vi "main.vi"() -> ()   [LabVIEW 2018]
uses:
  src/class/mqtt/mqttTypedef/mqttSubscribeCluster.ctl
  src/class/mqtt/mqttTypedef/mqttQOSlevel.ctl
  src/class/mqtt/mqttTypedef/mqttConnectionStatus.ctl
  src/class/mqtt/mqttTXqueue/mqttTXdataQueueFunction.ctl
  src/class/mqtt/mqttConfigFunction.ctl
  src/class/mqtt/mqttTXqueue/mqttRXsubscriptionEventFunction.ctl
  src/class/mqtt/mqttTypedef/mqttBroker.ctl
  src/class/mqtt/mqttTypedef/mqttConnectionFlags.ctl
  src/class/mqtt/mqttTypedef/mqttWillInformation.ctl
  src/class/mqtt/mqttTypedef/mqttConnectionMeta.ctl
  src/class/mqtt/mqtt.lvclass
panel:
  out "Connects":i32
  out "messageID":u16
  out "RX Value":string
  out "RX Topic":string
  in  "disconnect":bool
  out "sessionPresent":bool
  out "Connect Status":T1
  in  "connect":bool
  in  "subscriptionInfo":T2[](array[typedef])=[{"Topic"="channels/656489/subscribe/json/RVIIFSV5FO3T3HVM", "QoS"=enum."At most once"}]
  out "subscribeMessageID":u16 format="%02x"
  out "subscribeSuccess":bool
  out "valueSent":string="14:19:17.238_"
  out "publishMessageID":u16 format="%02x"
  in  "value":string="field1=16"
  in  "topic":string="channels/656489/publish/8Q3U783L32ZXTE0U"
  in  "quit":bool
  in  "subscribe":bool
  in  "publish":bool
  out "error out":errorcluster
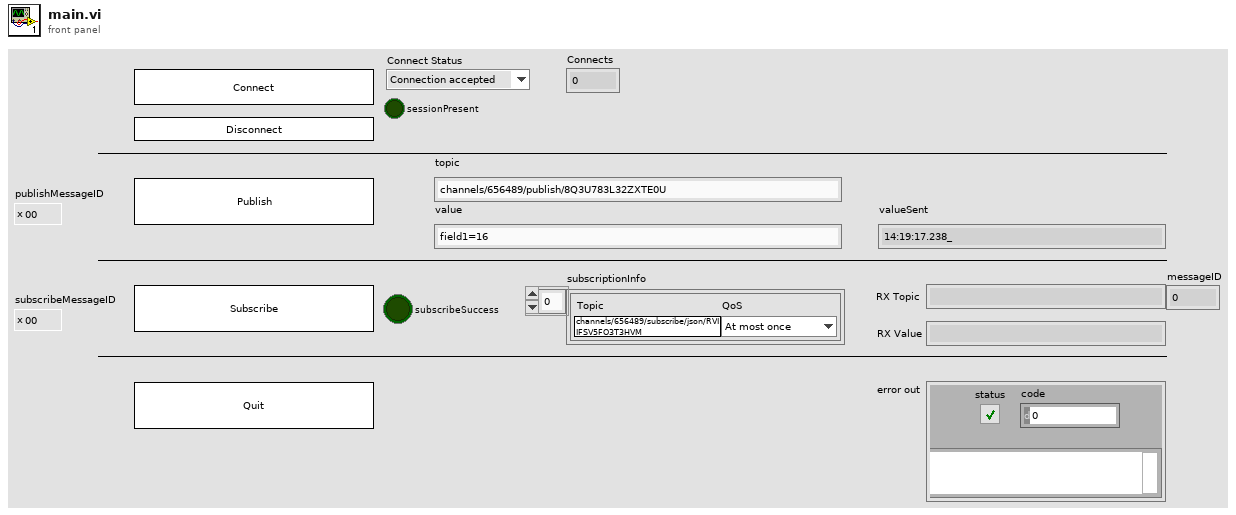
[diagram p1: front panel]
types:
  T1 = typedef "mqttConnectionStatus.ctl" = enum16{"Connection accepted", "Connection refused: unacceptable protocol version", "Connection refused: identifier rejected", "Connection refused: Server unavailable", "Connection refused: bad user name or password", "Connection refused: not authorized"}
  T2 = typedef "mqttSubscribeCluster.ctl" = cluster{"Topic":string, "QoS":T3}
  T3 = typedef "mqttQOSlevel.ctl" = enum8{"At most once", "At least once", "Exactly once", "Reserved"}
  T4 = typedef "mqttConnectionMeta.ctl" = cluster{"retain":bool, "duplicate":bool, "qos":T3}
  T5 = typedef "mqttWillInformation.ctl" = cluster{"User Name":string, "Password":string}
  T6 = typedef "mqttConnectionFlags.ctl" = cluster{"reserved":bool, "clean session":bool, "will flag":bool, "willQOS":enum8{"At most once", "At least once", "Exactly once", "Reserved"}, "will retain":bool, "password":bool, "user name":bool}
  T7 = typedef "mqttBroker.ctl" = cluster{"address":string, "port":u16, "connTimeout":i32, "writeTimeout":i32, "readTimeout":i32, "subTimeout":i32}
  T8 = typedef "mqttRXsubscriptionEventFunction.ctl" = enum16{"init", "deinit", "getEventRef", "event"}
  T9 = typedef "mqtt.lvclass/mqttConfigFunction.ctl" = enum16{"init", "deinit", "set", "get"}
  T10 = typedef "mqttTXdataQueueFunction.ctl" = enum16{"init", "deinit", "getQueue", "enqueue"}
  T11 = enum8{"Enabled", "Disabled", "Disabled and Grayed Out"}
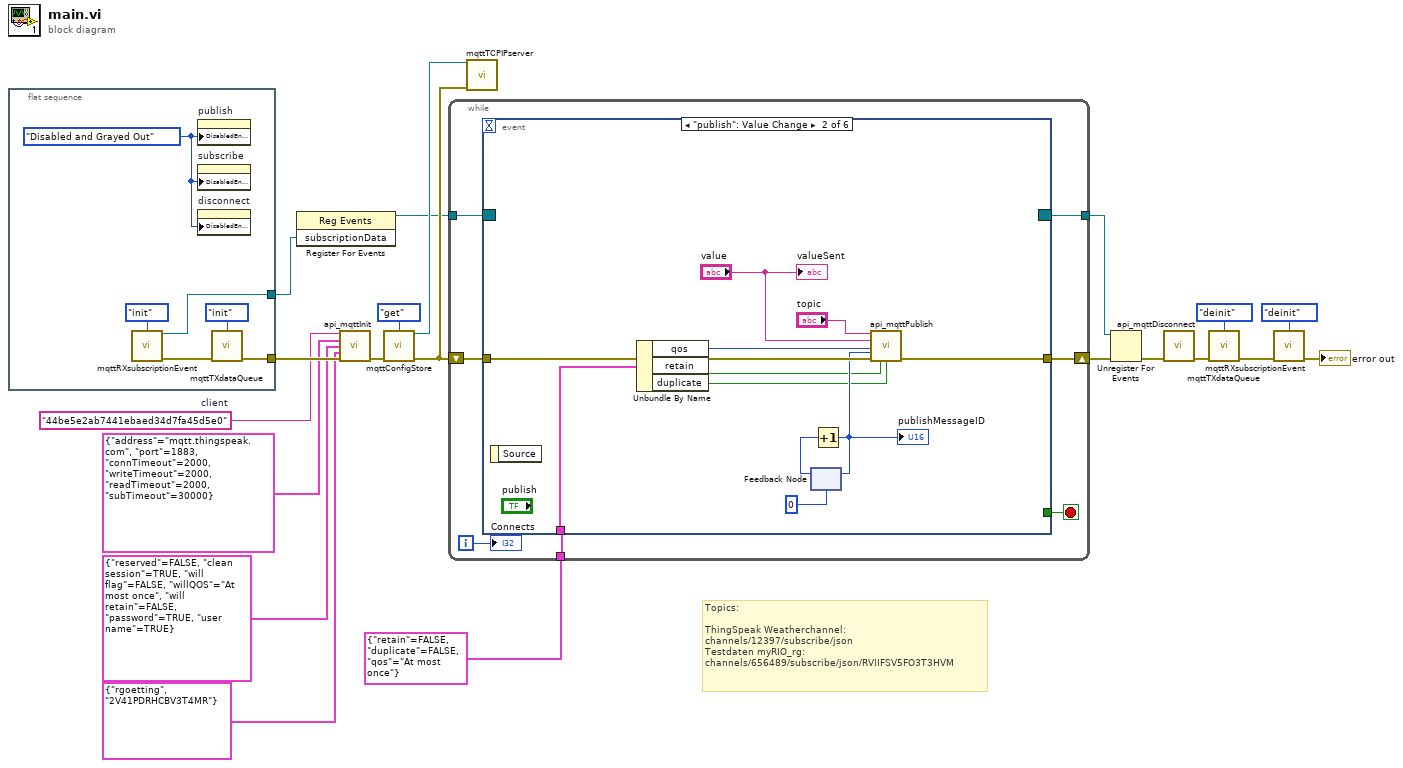
[diagram p0: block diagram]
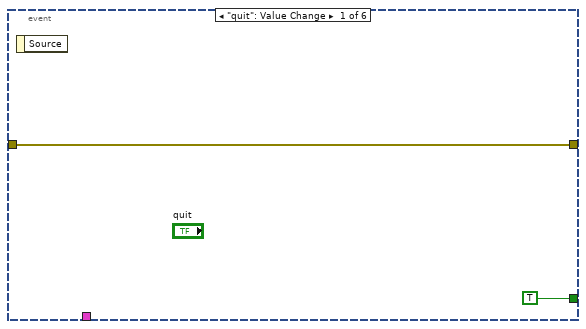
[diagram p2: hidden frame]
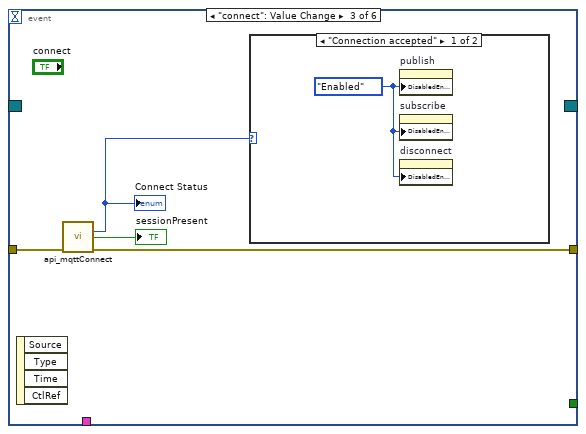
[diagram p3: hidden frame]
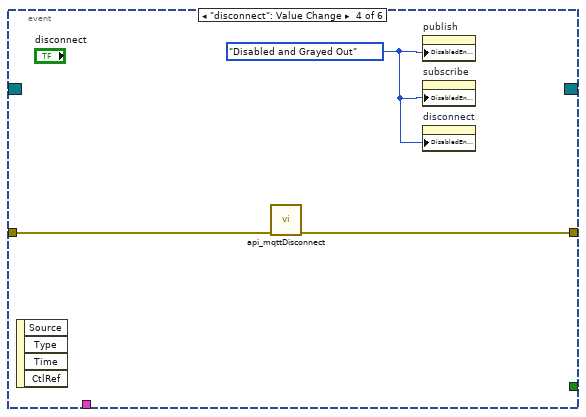
[diagram p5: hidden frame]
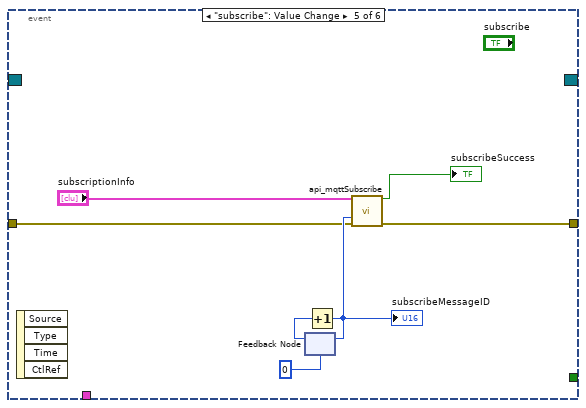
[diagram p6: hidden frame]
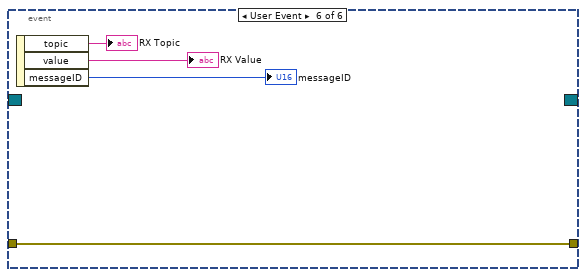
[diagram p7: hidden frame]
diagram:
  w5 = "44be5e2ab7441ebaed34d7fa45d5e0"  # client
  # "Topics:\n\nThingSpeak Weatherchannel:\nchannels/12397/subscribe/json\nTestdaten myRIO_rg:\nchannels/656489/subscribe/json/RVIIFSV5FO3T3HVM"
  n1 = flat-sequence {
    tunnel: [w25] -> w19
    tunnel: [w22] -> w13
    frame #0 {
      w21 = T11."Disabled and Grayed Out" ("Disabled")
      n2 = call "mqttRXsubscriptionEvent.vi"("function"=mqttRXsubscriptionEventFunction."init") -> ("subscriptionData"=w22:refnum<user-event>, "error out"=w24:errorcluster)  [unwired: 13 in]
      n3 = property on="publish" class="Bool"("DisabledEnum"=w21) -> ()  [unwired: 2 in, 2 out]
      n4 = property on="subscribe" class="Bool"("DisabledEnum"=w21) -> ()  [unwired: 2 in, 2 out]
      n5 = property on="disconnect" class="Bool"("DisabledEnum"=w21) -> ()  [unwired: 2 in, 2 out]
      n6 = call "mqttTXdataQueue.vi"("function"=mqttTXdataQueueFunction."init", "error in (no error)"=w24) -> ("error out"=w25:errorcluster)  [unwired: 12 in, 1 out]
    }
  }
  n7 = register-events(w13) -> (reference out=w12:refnum<event-registration>)  [unwired: 2 in, 1 out]
  n8 = call "api_mqttInit.vi"("client"=w5, "broker"=T7 {"address"="mqtt.thingspeak.com", "port"=1883, "connTimeout"=2000, "writeTimeout"=2000, "readTimeout"=2000, "subTimeout"=30000}, "connFlags"=T6 {"reserved"=FALSE, "clean session"=TRUE, "will flag"=FALSE, "willQOS"=enum."At most once", "will retain"=FALSE, "password"=TRUE, "user name"=TRUE}, "User Info"=T5 {"User Name"="rgoetting", "Password"="2V41PDRHCBV3T4MR"}, "error in (no error)"=w19) -> ("error out"=w17:errorcluster)  [unwired: 10 in]
  n9 = call "mqttConfigStore.vi"("function"=mqttConfigFunction."get", "error in (no error)"=w17) -> ("mqtt.lvclass out"=w16:refnum<class "mqtt.lvclass">, "error out"=w15:errorcluster)  [unwired: 12 in]
  n10 = while {
    shift-right: [w33] -> w8
    shift-left: w15 -> [w32]
    tunnel: w12 -> [w30]
    tunnel: [w28] -> w6
    tunnel: T4 {"retain"=FALSE, "duplicate"=FALSE, "qos"=enum."At most once"} ("connMeta") -> [w27]
    i -> [w29]
    stop <- w31 stop-if-true
    n11 = event shown="[1] \"publish\": Value Change" {
      selector: w30 -> [_ _ _ _ _ _]
      dyn-events: [_ _ _ _ _ _] -> w28
      timeout: _ -> [_ _ _ _ _ _]
      tunnel: [w34 w43 w49 w53 w57 w65] -> w33
      tunnel: w32 -> [w34 w44 w50 w54 w55 w65]
      tunnel: [TRUE _ _ _ _ _] -> w31
      tunnel: w27 -> [_ w37 _ _ _ _]
      event "quit": Value Change {
        n12 = event-data() -> ()  [unwired: 1 in, 1 out]
      }
      event "publish": Value Change {
        n13 = event-data() -> ()  [unwired: 1 in, 1 out]
        n14 = Unbundle By Name(w37) -> ("qos"=w40:T3, "retain"=w39:bool, "duplicate"=w38:bool)
        n15 = feedback #1(u16 0) -> (w45:u16)
        n16 = Increment(x=w45) -> (x+1=w42:u16)
        "publishMessageID" <- w42
        n17 = feedback-in #1(w42) -> ()
        n18 = call "api_mqttPublish.vi"("topic"="topic", "value"="value", "QoS (At most once)"=w40, "messageID"=w42, "error in (no error)"=w44, "retain(F)"=w39, "duplicate(F)"=w38) -> ("error out"=w43:errorcluster)  [unwired: 7 in, 1 out]
        "valueSent" <- "value"
      }
      event "connect": Value Change {
        n19 = event-data() -> ()  [unwired: 1 in, 4 out]
        n20 = call "api_mqttConnect.vi"("error in (no error)"=w50) -> ("connStatus"=w47:T1, "sessionPresent"=→"sessionPresent":bool, "error out"=w49:errorcluster)  [unwired: 11 in, 1 out]
        "Connect Status" <- w47
        n21 = case shown="\"Connection accepted\"" w47 {
          frame "Connection accepted" {
            w51 = T11."Enabled" ("Disabled")
            n22 = property on="publish" class="Bool"("DisabledEnum"=w51) -> ()  [unwired: 2 in, 2 out]
            n23 = property on="subscribe" class="Bool"("DisabledEnum"=w51) -> ()  [unwired: 2 in, 2 out]
            n24 = property on="disconnect" class="Bool"("DisabledEnum"=w51) -> ()  [unwired: 2 in, 2 out]
          }
          frame Default {
          }
        }
      }
      event "disconnect": Value Change {
        w52 = T11."Disabled and Grayed Out" ("Disabled")
        n25 = event-data() -> ()  [unwired: 1 in, 4 out]
        n26 = call "api_mqttDisconnect.vi"("error in (no error)"=w54) -> ("error out"=w53:errorcluster)  [unwired: 13 in, 1 out]
        n27 = property on="publish" class="Bool"("DisabledEnum"=w52) -> ()  [unwired: 2 in, 2 out]
        n28 = property on="subscribe" class="Bool"("DisabledEnum"=w52) -> ()  [unwired: 2 in, 2 out]
        n29 = property on="disconnect" class="Bool"("DisabledEnum"=w52) -> ()  [unwired: 2 in, 2 out]
      }
      event "subscribe": Value Change {
        n30 = event-data() -> ()  [unwired: 1 in, 4 out]
        n31 = feedback #2(u16 0) -> (w60:u16)
        n32 = Increment(x=w60) -> (x+1=w56:u16)
        "subscribeMessageID" <- w56
        n33 = feedback-in #2(w56) -> ()
        n34 = call "api_mqttSubscribe.vi"("subscriptionInfo"="subscriptionInfo", "messageID"=w56, "error in (no error)"=w55) -> ("success"=→"subscribeSuccess":bool, "error out"=w57:errorcluster)  [unwired: 11 in]
      }
      event User Event {
        n35 = event-data() -> ("topic"=→"RX Topic":string, "value"=→"RX Value":string, "messageID"=→"messageID":u16)  [unwired: 1 in]
      }
    }
    "Connects" <- w29
  }
  n36 = call "mqttTCPIPserver.vi"("mqtt.lvclass"=w16, "error in (no error)"=w15) -> ()  [unwired: 12 in, 2 out]
  n37 = Unregister For Events(event registration refnum=w6, error in=w8) -> (error out=w7:errorcluster)
  n38 = call "api_mqttDisconnect.vi"("error in (no error)"=w7) -> ("error out"=w14:errorcluster)  [unwired: 13 in, 1 out]
  n39 = call "mqttTXdataQueue.vi"("function"=mqttTXdataQueueFunction."deinit", "error in (no error)"=w14) -> ("error out"=w10:errorcluster)  [unwired: 12 in, 1 out]
  n40 = call "mqttRXsubscriptionEvent.vi"("function"=mqttRXsubscriptionEventFunction."deinit", "error in (no error)"=w10) -> ("error out"=→"error out":errorcluster)  [unwired: 12 in, 1 out]
